vi "AdjustXYZTclusterForPolarization.vi"(8 "TestZT":cluster{"Z mm":dbl, "Horizontal T deg":dbl}, 9 "Polarization":T1, 10 "Position, Horizontal":T2) -> (0 "TestZT out":cluster{"Z mm":dbl, "Horizontal T deg":dbl}, 2 "Position out":T2)   [LabVIEW 2018]
doc: "Positions are stored as X, Y, Z, T (deg) cluster (vector).\nT is stored in the configuration files as the Horizontal value.\nThis subvi rotates T 90 degrees to achieve an X, Y, Z, T for vertical polarization for the same XYZ position."
uses:
  PolarizationSelect.ctl
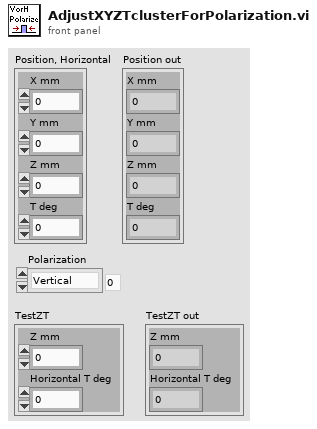
[diagram p1: front panel]
types:
  T1 = typedef "PolarizationSelect.ctl" = enum16{"Vertical", "Horizontal"}
  T2 = cluster{"X mm":dbl, "Y mm":dbl, "Z mm":dbl, "T deg":dbl}
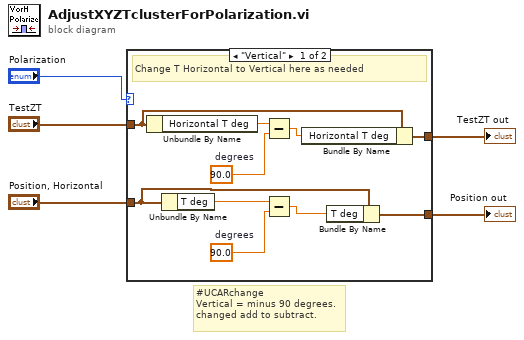
[diagram p0: block diagram]
diagram:
  # "#UCARchange \nVertical = minus 90 degrees.\nchanged add to subtract."
  n1 = case shown="\"Vertical\"" "Polarization" {
    tunnel: "Position, Horizontal" -> [w15 w17]
    tunnel: [w14 w17] -> w5
    tunnel: "TestZT" -> [w6 w16]
    tunnel: [w7 w16] -> w1
    frame "Vertical" {
      w8 = 90.0  # degrees
      w13 = 90.0  # degrees
      # "Change T Horizontal to Vertical here as needed"
      n2 = Unbundle By Name(w6) -> ("Horizontal T deg"=w9:dbl)
      n3 = Unbundle By Name(w15) -> ("T deg"=w12:dbl)
      n4 = Subtract(x=w9, y=w8) -> (x-y=w10:dbl)
      n5 = Subtract(x=w12, y=w13) -> (x-y=w11:dbl)
      n6 = Bundle By Name(cluster=w6, "Horizontal T deg"=w10) -> (w7:cluster{"Z mm":dbl, "Horizontal T deg":dbl})
      n7 = Bundle By Name(cluster=w15, "T deg"=w11) -> (w14:T2)
    }
    frame "Horizontal", Default {
      # "no change, Horizontal is baseline"
    }
  }
  "Position out" <- w5
  "TestZT out" <- w1
